vi "Arm v2.vi"() -> ()   [LabVIEW 2013]
uses:
  Globals/Homes.vi
  <vilib>/Rock Robotics/WPI/Joystick/WPI_JoystickGetSetRefNum.vi
  Robot Global Data.vi
  Globals/Auto.vi
  <vilib>/addons/control/pid/pid.llb/PID (DBL).vi
  Globals/Useful Values.vi
  <vilib>/addons/control/pid/NI_PID_pid.lvlib
panel:
  out "UP?":bool
  in  "PID gains DOWN":T1={"proportional gain (Kc)"=0.75, "integral time (Ti, min)"=0.0, "derivative time (Td, min)"=0.0} {"derivative time (Td, min)" format="%.3f"; "integral time (Ti, min)" format="%.3f"; "proportional gain (Kc)" format="%.3f"}
  out "Setpoint":dbl=0.808
  out "Motor Output":dbl=-0.22641594675000004
  in  "PID gains UP":T1={"proportional gain (Kc)"=6.0, "integral time (Ti, min)"=0.0, "derivative time (Td, min)"=0.0} {"derivative time (Td, min)" format="%.3f"; "integral time (Ti, min)" format="%.3f"; "proportional gain (Kc)" format="%.3f"}
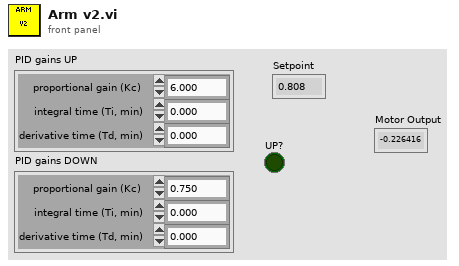
[diagram p1: front panel]
types:
  T1 = cluster{"proportional gain (Kc)":dbl, "integral time (Ti, min)":dbl, "derivative time (Td, min)":dbl}
  T2 = typedef "WPI_JoystickDevRef.ctl" = cluster{"Device":T3}
  T3 = typedef "WPI_JoystickDeviceEnum.ctl" = enum16{"USB 1", "USB 2", "USB 3", "USB 4", "Kinect 1", "Kinect 2"}
  T4 = typedef "WPI_AnalogChannelDevRef.ctl" = cluster{"DevStatus":errorcluster, "Analog Module":T5, "Analog Channel":T6}
  T5 = typedef "FPGA_TypedefAnalogModule.ctl" = enum16{"Analog Module 1", "Analog Module 2"}
  T6 = typedef "FPGA_AIChannel.ctl" = enum8{"AI 1", "AI 2", "AI 3", "AI 4", "AI 5", "AI 6", "AI 7", "AI 8", "Invalid"}
  T7 = typedef "WPI_DigitalInputDevRef.ctl" = cluster{"DevStatus":errorcluster, "DIO Channel":T8, "Digital Module":T9}
  T8 = typedef "FPGA_DIOChannel.ctl" = enum8{"DIO 1", "DIO 2", "DIO 3", "DIO 4", "DIO 5", "DIO 6", "DIO 7", "DIO 8", "DIO 9", "DIO 10", "DIO 11", "DIO 12", "DIO 13", "DIO 14", "Invalid"}
  T9 = typedef "FPGA_TypedefDigitalModule.ctl" = enum16{"Digital Module 1", "Digital Module 2"}
  T10 = typedef "WPI_MotorControlDeviceRef.ctl" = cluster{"DeviceStatus":errorcluster, "Type":enum16{"PWM", "CAN"}, "PWM":cluster{"Digital Module":T9, "PWM Channel":T11, "DeadBand":T12}, "CAN":cluster{"Device Number":u8, "Control Mode":T13, "Semaphore":T14, "Max Vout":dbl}, "Invert":bool, "TransformRef":T15, "InvTransformRef":T15}
  T11 = typedef "FPGA_DIOPWMChannel.ctl" = enum8{"PWM 1", "PWM 2", "PWM 3", "PWM 4", "PWM 5", "PWM 6", "PWM 7", "PWM 8", "PWM 9", "PWM 10", "Invalid"}
  T12 = typedef "WPI_PWMDeadband.ctl" = cluster{"Name":string, "maxPositivePwm":i32, "minPositivePwm":i32, "centerPwm":i32, "maxNegativePwm":i32, "minNegativePwm":i32, "angularRange":u16}
  T13 = typedef "WPI_CANJaguar_ControlMode.ctl" = enum8{"Percent VBus", "Current", "Speed", "Position", "Voltage"}
  T14 = typedef "Semaphore RefNum" = refnum<k1>
  T15 = typedef "WPI_PWMTransform_ConPane.ctl" = refnum<vi>
  T16 = typedef "WPI_DriverStationRobotMode2.ctl" = enum16{"Autonomous Disabled", "Autonomous Enabled", "Teleop Disabled", "Teleop Enabled", "Timeout", "Finish", "Test Disabled", "Test Enabled"}
  T17 = typedef "WPI_JoystickButtonState.ctl" = cluster{"Button 1":bool, "Button 2":bool, "Button 3":bool, "Button 4":bool, "Button 5":bool, "Button 6":bool, "Button 7":bool, "Button 8":bool, "Button 9":bool, "Button 10":bool, "Button 11":bool, "Button 12":bool}
  T18 = cluster{"axis 1 (x)":dbl, "axis 2 (y)":dbl, "axis 3 (throttle)":dbl, "axis 4":dbl, "axis 5":dbl, "axis 6":dbl}
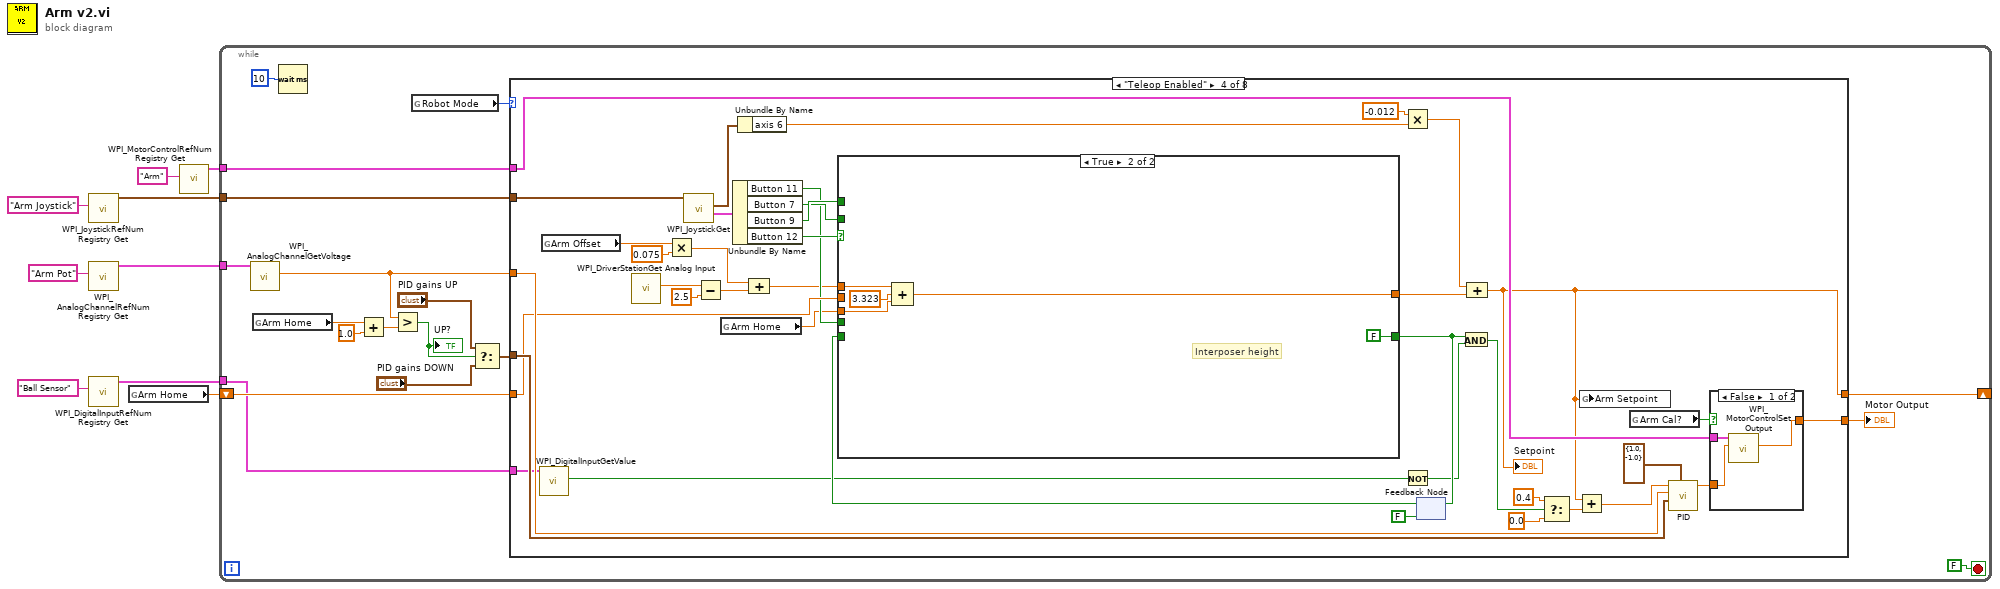
[diagram p0: block diagram]
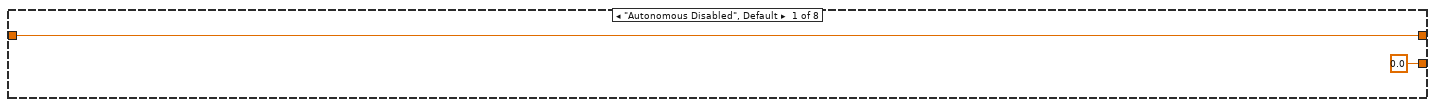
[diagram p2: hidden frame]
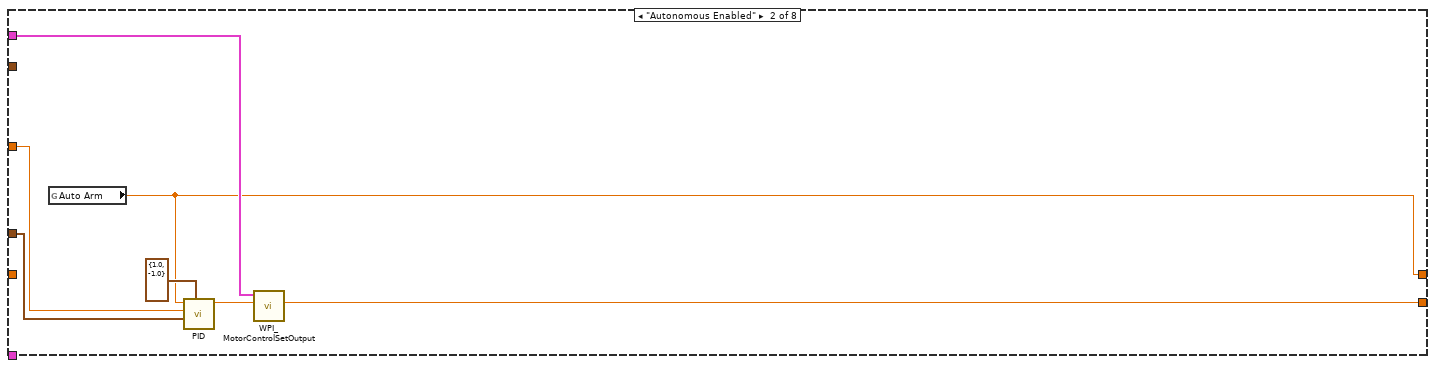
[diagram p3: hidden frame]
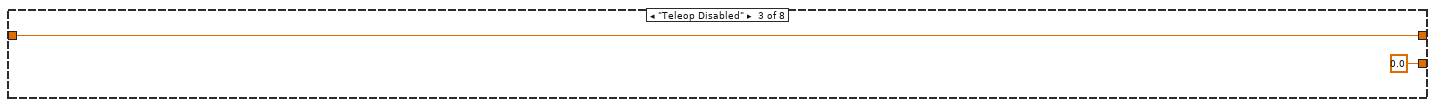
[diagram p4: hidden frame]
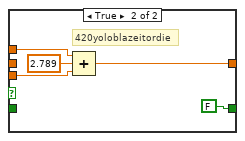
[diagram p6: hidden frame]
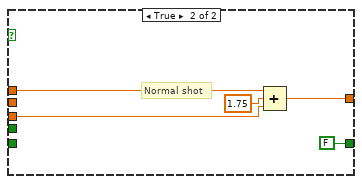
[diagram p7: hidden frame]
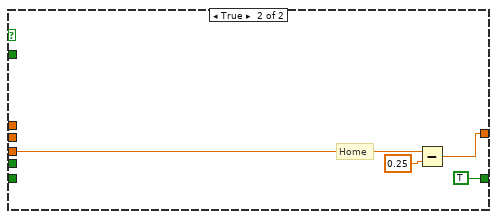
[diagram p8: hidden frame]
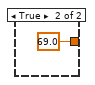
[diagram p9: hidden frame]
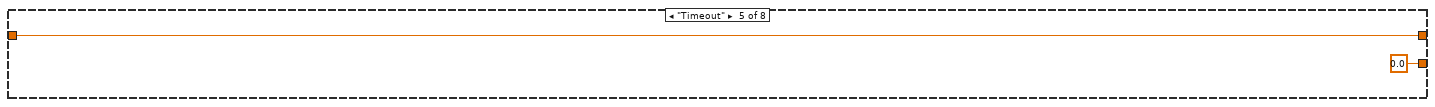
[diagram p10: hidden frame]
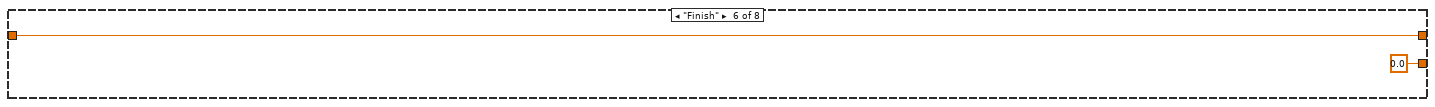
[diagram p11: hidden frame]
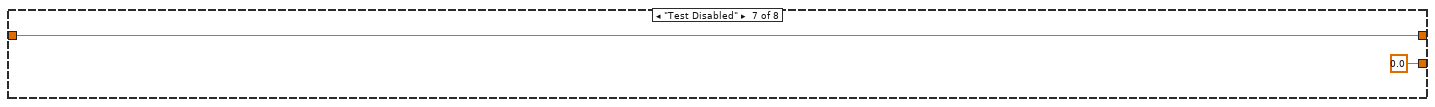
[diagram p12: hidden frame]
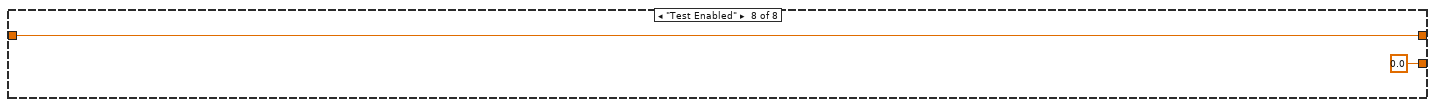
[diagram p13: hidden frame]
diagram:
  n1 = call <vilib>:"WPI_JoystickRefNum Registry Get.vi"("refnum name"="Arm Joystick") -> ("JoystickDevRef"=w4:T2)  [unwired: 9 in, 1 out]
  n2 = call <vilib>:"WPI_AnalogChannelRefNum Registry Get.vi"("refnum name"="Arm Pot") -> ("AIDeviceRef"=w9:T4)  [unwired: 9 in, 1 out]
  n3 = call <vilib>:"WPI_DigitalInputRefNum Registry Get.vi"("refnum name"="Ball Sensor") -> ("DigitalInputDevRef"=w2:T7)  [unwired: 9 in, 1 out]
  n4 = global read "Homes.vi" "Arm Home"() -> (w3:dbl)
  n5 = call <vilib>:"WPI_MotorControlRefNum Registry Get.vi"("refnum name"="Arm") -> ("MotorControlDevRef"=w6:T10)  [unwired: 9 in, 1 out]
  n6 = while {
    tunnel: w9 -> [w25]
    tunnel: w6 -> [w23]
    tunnel: w4 -> [w21]
    shift-right: [w20] -> _
    shift-left: w3 -> [w17]
    tunnel: w2 -> [w10]
    stop <- FALSE stop-if-true
    n7 = call <vilib>:"WPI_AnalogChannelGetVoltage.vi"("AIDeviceRef"=w25) -> ("Voltage"=w14:dbl)  [unwired: 8 in, 2 out]
    n8 = global read "Homes.vi" "Arm Home"() -> (w13:dbl)
    n9 = Wait (ms)(milliseconds to wait=u32 10) -> ()  [unwired: 1 out]
    n10 = Add(x=w13, y=1.0) -> (x+y=w11:dbl)
    n11 = Greater?(x=w14, y=w11) -> (0:w15:bool)
    "UP?" <- w15
    n12 = global read "Robot Global Data.vi" "Robot Mode"() -> (w24:T16)
    n13 = Select(t="PID gains UP", s=w15, f="PID gains DOWN") -> (s? t:f=w16:T1)
    n14 = case shown="\"Teleop Enabled\"" w24 {
      tunnel: w23 -> [_ w35 _ w71 _ _ _ _]
      tunnel: w14 -> [_ w33 _ w74 _ _ _ _]
      tunnel: [0.0 ("Motor Output") w34 0.0 ("Motor Output") w69 0.0 ("Motor Output") 0.0 ("Motor Output") 0.0 ("Motor Output") 0.0 ("Motor Output")] -> w22
      tunnel: w21 -> [_ _ _ w76 _ _ _ _]
      tunnel: w17 -> [w28 _ w37 w63 w127 w129 w131 w133]
      tunnel: [w28 w32 w37 w47 w127 w129 w131 w133] -> w20
      tunnel: w16 -> [_ w30 _ w73 _ _ _ _]
      tunnel: w10 -> [_ _ _ w55 _ _ _ _]
      frame "Autonomous Disabled", Default {
      }
      frame "Autonomous Enabled" {
        n15 = global read "Auto.vi" "Auto Arm"() -> (w32:dbl)
        n16 = call-poly <vilib>:"PID.vi"("output range"=cluster{"output high":dbl, "output low":dbl} {"output high"=1.0, "output low"=-1.0}, "PID gains"=w30, "process variable"=w33, "setpoint"=w32) -> ("output"=w31:dbl)  [unwired: 6 in, 1 out]
        n17 = call <vilib>:"WPI_MotorControlSetOutput.vi"("Output"=w31, "MotorControlDevRef"=w35) -> ("Motor Output"=w34:dbl)  [unwired: 7 in, 2 out]
      }
      frame "Teleop Disabled" {
      }
      frame "Teleop Enabled" {
        n18 = call <vilib>:"WPI_DigitalInputGetValue.vi"("DigitalInputDevRef"=w55) -> ("Value"=w52:bool)  [unwired: 8 in, 2 out]
        n19 = global read "Useful Values.vi" "Arm Offset"() -> (w43:dbl)
        n20 = call <vilib>:"WPI_DriverStationGet Analog Input.vi"() -> ("Analog 2 (V)"=w39:dbl)  [unwired: 8 in, 3 out]
        n21 = Multiply(x=w43, y=0.075) -> (x*y=w45:dbl)
        n22 = call <vilib>:"WPI_JoystickGet.vi"("JoystickDevRef"=w76) -> ("Buttons"=w75:T17, "Axes"=w68:T18)  [unwired: 4 in, 1 out]
        n23 = Subtract(x=w39, y=2.5) -> (x-y=w41:dbl)
        n24 = global read "Homes.vi" "Arm Home"() -> (w59:dbl)
        n25 = Unbundle By Name(w75) -> ("Button 11"=w60:bool, "Button 7"=w64:bool, "Button 9"=w65:bool, "Button 12"=w66:bool)
        n26 = Unbundle By Name(w68) -> ("axis 6"=w61:dbl)
        n27 = Compound Arithmetic op=ADD(w45, w41) -> (w40:dbl)
        n28 = Multiply(x=-0.012, y=w61) -> (x*y=w58:dbl)
        n29 = Not(x=w52) -> (.not. x?=w50:bool)
        n30 = feedback #1(FALSE) -> (w57:bool)
        n31 = case shown="True" w66 {
          tunnel: w63 -> [w81 _]
          tunnel: [w84 w120] -> w62
          tunnel: w59 -> [w85 w121]
          tunnel: w40 -> [w82 w122]
          tunnel: w65 -> [w86 _]
          tunnel: w64 -> [w83 _]
          tunnel: w60 -> [w80 _]
          tunnel: [w79 FALSE] -> w51
          tunnel: w57 -> [w78 _]
          frame False {
            n32 = case shown="False" w86 {
              tunnel: w85 -> [w92 w117]
              tunnel: [w91 w115] -> w84
              tunnel: w83 -> [w94 _]
              tunnel: w82 -> [w93 _]
              tunnel: w81 -> [w90 _]
              tunnel: w80 -> [w89 _]
              tunnel: [w88 TRUE] -> w79
              tunnel: w78 -> [w87 _]
              frame False {
                n33 = case shown="False" w94 {
                  tunnel: w93 -> [w100 w113]
                  tunnel: w92 -> [w101 w112]
                  tunnel: [w99 w110] -> w91
                  tunnel: w90 -> [w98 _]
                  tunnel: w89 -> [w97 _]
                  tunnel: [w96 FALSE] -> w88
                  tunnel: w87 -> [w95 _]
                  frame False {
                    n34 = case shown="False" w97 {
                      tunnel: w101 -> [_ w108]
                      tunnel: w100 -> [_ w107]
                      tunnel: [w103 w105] -> w99
                      tunnel: w98 -> [w103 _]
                      tunnel: [w102 FALSE] -> w96
                      tunnel: w95 -> [w102 _]
                      frame False {
                      }
                      frame True {
                        # "420yoloblazeitordie"
                        n35 = Compound Arithmetic op=ADD(w107, 2.789 ("value"), w108) -> (w105:dbl)
                      }
                    }
                  }
                  frame True {
                    # "Normal shot"
                    n36 = Compound Arithmetic op=ADD(w113, 1.75 ("value"), w112) -> (w110:dbl)
                  }
                }
              }
              frame True {
                # "Home"
                n37 = Subtract(x=w117, y=0.25) -> (x-y=w115:dbl)
              }
            }
          }
          frame True {
            # "Interposer height"
            n38 = Compound Arithmetic op=ADD(w122, 3.323 ("value"), w121) -> (w120:dbl)
          }
        }
        n39 = feedback-in #1(w51) -> ()
        n40 = And(x=w51, y=w50) -> (x .and. y?=w49:bool)
        n41 = Compound Arithmetic op=ADD(w58, w62) -> (w47:dbl)
        "Setpoint" <- w47
        n42 = Select(t=0.4, s=w49, f=0.0) -> (s? t:f=w46:dbl)
        n43 = Add(x=w47, y=w46) -> (x+y=w48:dbl)
        n44 = global write "Useful Values.vi" "Arm Setpoint"(w47) -> ()
        n45 = global read "Useful Values.vi" "Arm Cal?"() -> (w72:bool)
        n46 = call-poly <vilib>:"PID.vi"("output range"=cluster{"output high":dbl, "output low":dbl} {"output high"=1.0, "output low"=-1.0}, "PID gains"=w73, "process variable"=w74, "setpoint"=w48) -> ("output"=w70:dbl)  [unwired: 6 in, 1 out]
        n47 = case shown="False" w72 {
          tunnel: w71 -> [w125 _]
          tunnel: w70 -> [w124 _]
          tunnel: [w123 69.0 ("Motor Output")] -> w69
          frame False {
            n48 = call <vilib>:"WPI_MotorControlSetOutput.vi"("Output"=w124, "MotorControlDevRef"=w125) -> ("Motor Output"=w123:dbl)  [unwired: 7 in, 2 out]
          }
          frame True {
          }
        }
      }
      frame "Timeout" {
      }
      frame "Finish" {
      }
      frame "Test Disabled" {
      }
      frame "Test Enabled" {
      }
    }
    "Motor Output" <- w22
  }
